vi "Set Timing.vi"(8 "error in (no error)":errorcluster, 9 "Timing Engine":T1=enum."Low Speed", 10 "Timing Info":T2, 11 "Cfg Grandmaster in":refnum<class "Cfg Grandmaster.lvclass">) -> (0 "error out":errorcluster, 3 "Cfg Grandmaster out":refnum<class "Cfg Grandmaster.lvclass">)   [LabVIEW 2018, in "Configuration Grandmaster.lvlib" / "Cfg Grandmaster.lvclass"]
uses:
  Cfg Grandmaster.lvclass
  Common/Controls/Group Timing Info.ctl
  Common/Controls/TE_Designator.ctl
  Cfg Grandmaster.lvclass/Cfg Grandmaster.ctl
  Class Chassis Cfg/ChassisCfg.lvclass
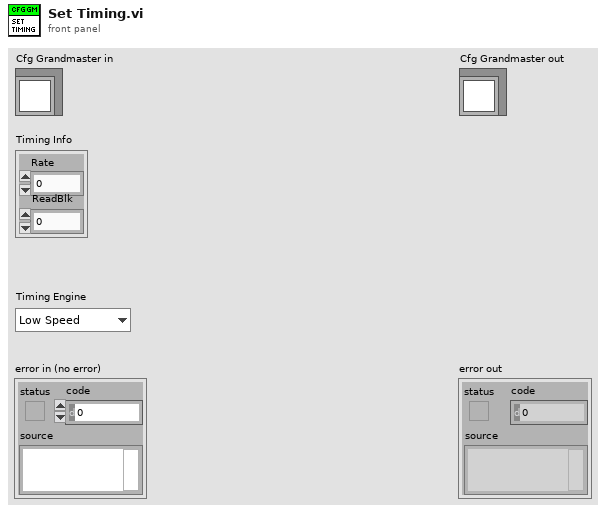
[diagram p1: front panel]
types:
  T1 = typedef "TE_Designator.ctl" = enum16{"High Speed", "Low Speed"}
  T2 = typedef "Group Timing Info.ctl" = cluster{"Rate":dbl, "ReadBlk":i32}
  T3 = typedef "ge_Cfg wChassis.ctl" = cluster{"Chassis BOM":refnum<class "Chassis BOM.lvclass">, "Chassis Cfg":refnum<class "ChassisCfg.lvclass">, "Chassis Tasks":refnum<class "Chassis Tasks.lvclass">, "HW Error":bool, "Unsvd Chgs?":bool}
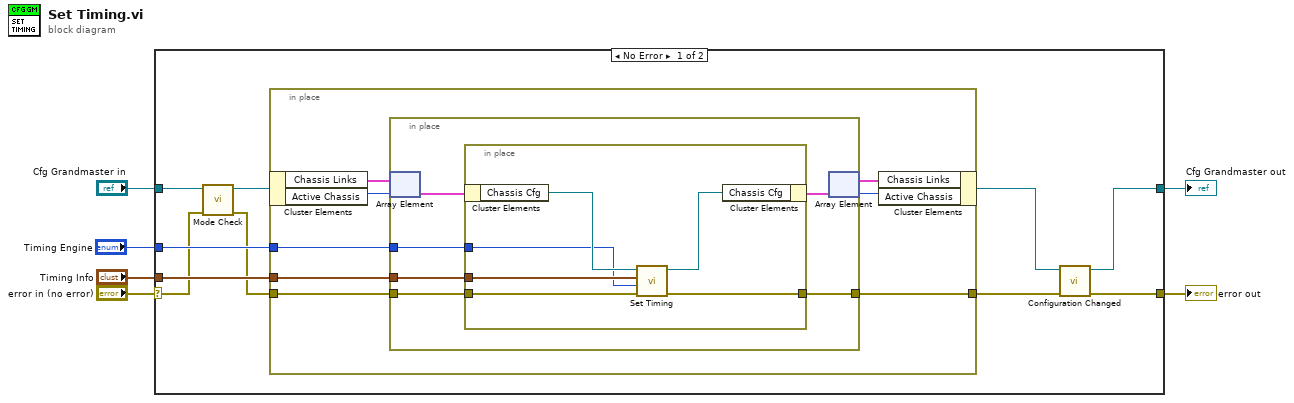
[diagram p0: block diagram]
diagram:
  n1 = case shown="No Error" "error in (no error)" {
    selector: "error in (no error)" -> [w12 w38]
    tunnel: [w9 w38] -> w5
    tunnel: [w7 w37] -> w3
    tunnel: "Cfg Grandmaster in" -> [w14 w37]
    tunnel: "Timing Engine" -> [w16 _]
    tunnel: "Timing Info" -> [w15 _]
    frame No Error {
      n2 = call "Mode Check.vi"("error in (no error)"=w12, "Cfg Grandmaster in"=w14) -> ("error out"=w11:errorcluster, "Cfg Grandmaster out"=w13:refnum<class "Cfg Grandmaster.lvclass">)  [unwired: 8 in]
      n3 = in-place {
        in-place-border: [w22] -> w10
        in-place-border: w11 -> [w21]
        in-place-border: w16 -> [w20]
        in-place-border: w15 -> [w19]
        n4 = in-place-cluster #1(w13) -> ("Chassis Links"=w24:T3[], "Active Chassis"=w18:i32)
        n5 = in-place {
          in-place-border: [w30] -> w22
          in-place-border: w19 -> [w27]
          in-place-border: w21 -> [w26]
          in-place-border: w20 -> [w25]
          n6 = in-place-array #2(w24, w18) -> (w29:T3)
          n7 = in-place {
            in-place-border: [w36] -> w30
            in-place-border: w27 -> [w32]
            in-place-border: w26 -> [w35]
            in-place-border: w25 -> [w31]
            n8 = in-place-cluster #3(w29) -> ("Chassis Cfg"=w34:refnum<class "ChassisCfg.lvclass">)
            n9 = call "Set Timing.vi"("error in (no error)"=w35, "Timing Engine"=w31, "TimingCfg"=w32, "Chassis Cfg"=w34) -> ("error out"=w36:errorcluster, "Chassis Cfg"=w33:refnum<class "ChassisCfg.lvclass">)  [unwired: 6 in]
            n10 = in-place-cluster #3("Chassis Cfg"=w33) -> (w28:T3)
          }
          n11 = in-place-array #2(w28) -> (w23:T3[], w17:i32)
        }
        n12 = in-place-cluster #1("Chassis Links"=w23, "Active Chassis"=w17) -> (w8:refnum<class "Cfg Grandmaster.lvclass">)
      }
      n13 = call "Configuration Changed.vi"("error in (no error)"=w10, "Cfg Grandmaster in"=w8) -> ("error out"=w9:errorcluster, "Cfg Grandmaster out"=w7:refnum<class "Cfg Grandmaster.lvclass">)  [unwired: 8 in]
    }
    frame Error {
    }
  }
  "error out" <- w5
  "Cfg Grandmaster out" <- w3
